vi "test_read-nmea-data2.vi"() -> ()   [LabVIEW 2019] (continued)
248,29,06,64,051,31,6*6C\n\t\n15:15:10.47\tF9P\t$GPGSV,3,2,09,09,44,072,30,12,23,275,18,17,31,154,18,19,51,157,,6*6D\n\t\n15:15:10.49\tF9P\t$GPGSV,3,3,09,25,12,305,,6*58\n\t\n15:15:10.51\tF9P\t$GLGSV,2,1,08,69,10,031,25,70,70,037,29,71,54,207,37,72,05,210,,1*72\n\t\n15:15:10.53\tF9P\t$GLGSV,2,2,08,77,01,324,,84,19,123,16,85,69,072,34,86,38,331,,1*73\n\t\n15:15:10.55\tF9P\t$GLGSV,2,1,08,69,10,031,19,70,70,037,,71,54,207,29,72,05,210,,3*7B\n\t\n15:15:10.57\tF9P\t$GLGSV,2,2,08,77,01,324,,84,19,123,19,85,69,072,27,86,38,331,,3*7C\n\t\n15:15:10.59\tF9P\t$GAGSV,2,1,08,02,08,296,10,04,67,115,41,09,33,193,23,11,72,001,30,7*7F\n\t\n15:15:10.61\tF9P\t$GAGSV,2,2,08,12,39,103,22,19,25,045,28,25,08,248,,36,27,309,22,7*7F\n\t\n15:15:10.63\tF9P\t$GAGSV,2,1,08,02,08,296,,04,67,115,,09,33,193,,11,72,001,,2*7C\n\t\n15:15:10.65\tF9P\t$GAGSV,2,2,08,12,39,103,,19,25,045,20,25,08,248,,36,27,309,,2*72\n\t\n15:15:10.67\tF9P\t$GBGSV,2,1,06,07,,,21,11,48,133,38,14,87,101,28,28,,,24,1*7D\n\t\n15:15:10.69\tF9P\t$GBGSV,2,2,06,33,62,220,29,34,,,28,1*42\n\t\n15:15:10.71\tF9P\t$GBGSV,1,1,03,11,48,133,,14,87,101,28,33,62,220,,3*4E\n\t\n15:15:10.73\tF9P\t$GNGLL,3723.60078,N,12656.94421,E,061512.00,A,A*76\n\t\n15:15:10.75\tF9P\t\t\n15:15:10.77\tF9P\t\t\n15:15:10.79\tF9P\t\t\n15:15:10.81\tF9P\t\t\n15:15:10.83\tF9P\t\t\n15:15:10.85\tF9P\t\t\n15:15:10.87\tF9P\t\t\n15:15:10.89\tF9P\t\t\n15:15:10.91\tF9P\t\t\n15:15:10.93\tF9P\t\t\n15:15:10.95\tF9P\t\t\n15:15:10.97\tF9P\t\t\n15:15:10.99\tF9P\t\t\n15:15:11.01\tF9P\t\t\n15:15:11.03\tF9P\t\t\n15:15:11.05\tF9P\t\t\n15:15:11.07\tF9P\t\t\n15:15:11.09\tF9P\t\t\n15:15:11.11\tF9P\t\t\n15:15:11.13\tF9P\t\t\n15:15:11.15\tF9P\t\t\n15:15:11.17\tF9P\t\t\n15:15:11.19\tF9P\t\t\n15:15:11.21\tF9P\t\t\n15:15:11.23\tF9P\t\t\n15:15:11.25\tF9P\t$GNRMC,061513.00,A,3723.60061,N,12656.94322,E,2.887,256.84,250720,,,A,V*0C\n\t\n15:15:11.27\tF9P\t$GNVTG,256.84,T,,M,2.887,N,5.347,K,A*2E\n\t\n15:15:11.29\tF9P\t$GNGGA,061513.00,3723.60061,N,12656.94322,E,1,12,0.71,45.1,M,18.5,M,,*77\n\t\n15:15:11.31\tF9P\t$GNGSA,A,3,12,06,19,05,17,09,04,02,,,,,1.23,0.71,1.00,1*07\n\t\n15:15:11.33\tF9P\t$GNGSA,A,3,85,70,71,84,,,,,,,,,1.23,0.71,1.00,2*05\n\t\n15:15:11.35\tF9P\t$GNGSA,A,3,36,19,11,04,09,12,,,,,,,1.23,0.71,1.00,3*07\n\t\n15:15:11.37\tF9P\t$GNGSA,A,3,14,11,33,,,,,,,,,,1.23,0.71,1.00,4*06\n\t\n15:15:11.39\tF9P\t$GPGSV,3,1,09,02,56,320,26,04,17,043,29,05,38,248,35,06,64,051,41,1*66\n\t\n15:15:11.41\tF9P\t$GPGSV,3,2,09,09,44,072,39,12,23,275,27,17,31,154,26,19,51,157,27,1*67\n\t\n15:15:11.43\tF9P\t$GPGSV,3,3,09,25,12,305,08,1*57\n\t\n15:15:11.45\tF9P\t$GPGSV,3,1,09,02,56,320,,04,17,043,21,05,38,248,29,06,64,051,31,6*67\n\t\n15:15:11.47\tF9P\t$GPGSV,3,2,09,09,44,072,30,12,23,275,18,17,31,154,17,19,51,157,,6*62\n\t\n15:15:11.49\tF9P\t$GPGSV,3,3,09,25,12,305,,6*58\n\t\n15:15:11.51\tF9P\t$GLGSV,2,1,08,69,10,031,26,70,70,037,29,71,54,207,29,72,05,210,,1*7E\n\t\n15:15:11.53\tF9P\t$GLGSV,2,2,08,77,01,324,,84,19,123,17,85,69,072,34,86,38,331,,1*72\n\t\n15:15:11.55\tF9P\t$GLGSV,2,1,08,69,10,031,19,70,70,037,,71,54,207,28,72,05,210,,3*7A\n\t\n15:15:11.57\tF9P\t$GLGSV,2,2,08,77,01,324,,84,19,123,20,85,69,072,26,86,38,331,,3*77\n\t\n15:15:11.59\tF9P\t$GAGSV,2,1,08,02,08,296,10,04,67,115,40,09,33,193,23,11,72,001,25,7*7A\n\t\n15:15:11.61\tF9P\t$GAGSV,2,2,08,12,39,103,22,19,25,045,29,25,08,248,,36,27,309,29,7*75\n\t\n15:15:11.63\tF9P\t$GAGSV,2,1,08,02,08,296,,04,67,115,29,09,33,193,,11,72,001,,2*77\n\t\n15:15:11.65\tF9P\t$GAGSV,2,2,08,12,39,103,,19,25,045,19,25,08,248,,36,27,309,28,2*72\n\t\n15:15:11.67\tF9P\t$GBGSV,2,1,06,07,,,21,11,48,133,26,14,87,101,28,28,,,24,1*72\n\t\n15:15:11.69\tF9P\t$GBGSV,2,2,06,33,62,220,33,34,,,28,1*49\n\t\n15:15:11.71\tF9P\t$GBGSV,1,1,03,11,48,133,,14,87,101,28,33,62,220,,3*4E\n\t\n15:15:11.73\tF9P\t$GNGLL,3723.60061,N,12656.94322,E,061513.00,A,A*7B\n\t\n15:15:11.75\tF9P\t\t\n15:15:11.77\tF9P\t\t\n15:15:11.79\tF9P\t\t\n15:15:11.81\tF9P\t\t\n15:15:11.83\tF9P\t\t\n15:15:11.85\tF9P\t\t\n15:15:11.87\tF9P\t\t\n15:15:11.89\tF9P\t\t\n15:15:11.91\tF9P\t\t\n15:15:11.93\tF9P\t\t\n15:15:11.95\tF9P\t\t\n15:15:11.97\tF9P\t\t\n15:15:11.99\tF9P\t\t\n15:15:12.01\tF9P\t\t\n15:15:12.03\tF9P\t\t\n15:15:12.05\tF9P\t\t\n15:15:12.07\tF9P\t\t\n15:15:12.09\tF9P\t\t\n15:15:12.11\tF9P\t\t\n15:15:12.13\tF9P\t\t\n15:15:12.15\tF9P\t\t\n15:15:12.17\tF9P\t\t\n15:15:12.19\tF9P\t\t\n15:15:12.21\tF9P\t\t\n15:15:12.23\tF9P\t$GNRMC,061514.00,A,3723.60011,N,12656.94253,E,2.747,249.72,250720,,,A,V*0F\n\t\n15:15:12.25\tF9P\t$GNVTG,249.72,T,,M,2.747,N,5.087,K,A*25\n\t\n15:15:12.27\tF9P\t$GNGGA,061514.00,3723.60011,N,12656.94253,E,1,12,0.75,44.4,M,18.5,M,,*70\n\t\n15:15:12.29\tF9P\t$GNGSA,A,3,12,06,19,05,17,09,04,02,,,,,1.25,0.75,1.01,1*04\n\t\n15:15:12.31\tF9P\t$GNGSA,A,3,85,70,71,84,,,,,,,,,1.25,0.75,1.01,2*06\n\t\n15:15:12.33\tF9P\t$GNGSA,A,3,36,19,11,04,09,12,,,,,,,1.25,0.75,1.01,3*04\n\t\n15:15:12.35\tF9P\t$GNGSA,A,3,14,11,33,,,,,,,,,,1.25,0.75,1.01,4*05\n\t\n15:15:12.37\tF9P\t$GPGSV,3,1,09,02,56,320,26,04,17,043,29,05,38,248,31,06,64,051,40,1*63\n\t\n15:15:12.39\tF9P\t$GPGSV,3,2,09,09,44,072,41,12,23,275,26,17,31,154,27,19,51,157,31,1*6F\n\t\n15:15:12.41\tF9P\t$GPGSV,3,3,09,25,12,305,,1*5F\n\t\n15:15:12.43\tF9P\t$GPGSV,3,1,09,02,56,320,,04,17,043,19,05,38,248,28,06,64,051,32,6*6E\n\t\n15:15:12.45\tF9P\t$GPGSV,3,2,09,09,44,072,29,12,23,275,19,17,31,154,17,19,51,157,,6*6B\n\t\n15:15:12.47\tF9P\t$GPGSV,3,3,09,25,12,305,,6*58\n\t\n15:15:12.49\tF9P\t$GLGSV,2,1,08,69,10,031,31,70,70,037,32,71,54,207,28,72,05,210,,1*73\n\t\n15:15:12.51\tF9P\t$GLGSV,2,2,08,77,01,324,,84,19,123,18,85,69,072,40,86,38,331,,1*7E\n\t\n15:15:12.53\tF9P\t$GLGSV,2,1,08,69,10,031,18,70,70,037,,71,54,207,27,72,05,210,,3*74\n\t\n15:15:12.55\tF9P\t$GLGSV,2,2,08,77,01,324,,84,19,123,21,85,69,072,26,86,38,331,,3*76\n\t\n15:15:12.57\tF9P\t$GAGSV,2,1,08,02,08,296,11,04,67,115,37,09,33,193,30,11,72,001,24,7*78\n\t\n15:15:12.59\tF9P\t$GAGSV,2,2,08,12,39,103,29,19,25,045,33,25,08,248,,36,27,309,27,7*7B\n\t\n15:15:12.61\tF9P\t$GAGSV,2,1,08,02,08,296,,04,67,115,,09,33,193,,11,72,001,,2*7C\n\t\n15:15:12.63\tF9P\t$GAGSV,2,2,08,12,39,103,,19,25,045,19,25,08,248,,36,27,309,25,2*7F\n\t\n15:15:12.65\tF9P\t$GBGSV,2,1,06,07,,,21,11,48,133,27,14,87,101,32,28,,,25,1*79\n\t\n15:15:12.67\tF9P\t$GBGSV,2,2,06,33,62,220,35,34,,,27,1*40\n\t\n15:15:12.69\tF9P\t$GBGSV,1,1,03,11,48,133,,14,87,101,32,33,62,220,,3*45\n\t\n15:15:12.71\tF9P\t$GNGLL,3723.60011,N,12656.94253,E,061514.00,A,A*7C\n\t\n15:15:12.73\tF9P\t\t\n15:15:12.75\tF9P\t\t\n15:15:12.77\tF9P\t\t\n15:15:12.79\tF9P\t\t\n15:15:12.81\tF9P\t\t\n15:15:12.83\tF9P\t\t\n15:15:12.85\tF9P\t\t\n15:15:12.87\tF9P\t\t\n15:15:12.89\tF9P\t\t\n15:15:12.91\tF9P\t\t\n15:15:12.93\tF9P\t\t\n15:15:12.95\tF9P\t\t\n15:15:12.97\tF9P\t\t\n15:15:12.99\tF9P\t\t\n15:15:13.01\tF9P\t\t\n15:15:13.03\tF9P\t\t\n15:15:13.05\tF9P\t\t\n15:15:13.07\tF9P\t\t\n15:15:13.09\tF9P\t\t\n15:15:13.11\tF9P\t\t\n15:15:13.13\tF9P\t\t\n15:15:13.15\tF9P\t\t\n15:15:13.17\tF9P\t\t\n15:15:13.19\tF9P\t\t\n15:15:13.21\tF9P\t\t\n15:15:13.23\tF9P\t$GNRMC,061515.00,A,3723.59977,N,12656.94169,E,2.605,246.33,250720,,,A,V*0A\n\t\n15:15:13.25\tF9P\t$GNVTG,246.33,T,,M,2.605,N,4.825,K,A*29\n\t\n15:15:13.27\tF9P\t$GNGGA,061515.00,3723.59977,N,12656.94169,E,1,12,0.72,44.4,M,18.5,M,,*7F\n\t\n15:15:13.29\tF9P\t$GNGSA,A,3,12,06,19,05,17,09,04,02,,,,,1.24,0.72,1.00,1*03\n\t\n15:15:13.31\tF9P\t$GNGSA,A,3,85,70,71,84,,,,,,,,,1.24,0.72,1.00,2*01\n\t\n15:15:13.33\tF9P\t$GNGSA,A,3,36,19,11,04,09,12,,,,,,,1.24,0.72,1.00,3*03\n\t\n15:15:13.35\tF9P\t$GNGSA,A,3,14,11,33,,,,,,,,,,1.24,0.72,1.00,4*02\n\t\n15:15:13.37\tF9P\t$GPGSV,3,1,09,02,56,320,26,04,17,043,28,05,38,248,34,06,64,051,34,1*64\n\t\n15:15:13.39\tF9P\t$GPGSV,3,2,09,09,44,072,42,12,23,275,27,17,31,154,27,19,51,157,39,1*65\n\t\n15:15:13.41\tF9P\t$GPGSV,3,3,09,25,12,305,,1*5F\n\t\n15:15:13.43\tF9P\t$GPGSV,3,1,09,02,56,320,,04,17,043,20,05,38,248,27,06,64,051,31,6*68\n\t\n15:15:13.45\tF9P\t$GPGSV,3,2,09,09,44,072,31,12,23,275,18,17,31,154,17,19,51,157,,6*63\n\t\n15:15:13.47\tF9P\t$GPGSV,3,3,09,25,12,305,,6*58\n\t\n15:15:13.49\tF9P\t$GLGSV,2,1,08,69,10,031,31,70,70,037,25,71,54,207,36,72,05,210,,1*7A\n\t\n15:15:13.51\tF9P\t$GLGSV,2,2,08,77,01,324,,84,19,123,18,85,69,072,36,86,38,331,,1*7F\n\t\n15:15:13.53\tF9P\t$GLGSV,2,1,08,69,10,031,17,70,70,037,,71,54,207,25,72,05,210,,3*79\n\t\n15:15:13.55\tF9P\t$GLGSV,2,2,08,77,01,324,,84,19,123,19,85,69,072,27,86,38,331,,3*7C\n\t\n15:15:13.57\tF9P\t$GAGSV,2,1,08,02,08,296,09,04,67,115,37,09,33,193,30,11,72,001,25,7*70\n\t\n15:15:13.59\tF9P\t$GAGSV,2,2,08,12,39,103,27,19,25,045,28,25,08,248,,36,27,309,25,7*7D\n\t\n15:15:13.61\tF9P\t$GAGSV,2,1,08,02,08,296,,04,67,115,,09,33,193,,11,72,001,,2*7C\n\t\n15:15:13.63\tF9P\t$GAGSV,2,2,08,12,39,103,,19,25,045,20,25,08,248,,36,27,309,23,2*73\n\t\n15:15:13.65\tF9P\t$GBGSV,2,1,06,07,,,21,11,48,133,32,14,87,101,32,28,,,31,1*78\n\t\n15:15:13.67\tF9P\t$GBGSV,2,2,06,33,62,220,36,34,,,27,1*43\n\t\n15:15:13.69\tF9P\t$GBGSV,1,1,03,11,48,133,,14,87,101,29,33,62,220,,3*4F\n\t\n15:15:13.71\tF9P\t$GNGLL,3723.59977,N,12656.94169,E,061515.00,A,A*74\n\t\n15:15:13.73\tF9P\t\t\n15:15:13.75\tF9P\t\t\n15:15:13.77\tF9P\t\t\n15:15:13.79\tF9P\t\t\n15:15:13.81\tF9P\t\t\n15:15:13.83\tF9P\t\t\n15:15:13.85\tF9P\t\t\n15:15:13.87\tF9P\t\t\n15:15:13.89\tF9P\t\t\n15:15:13.91\tF9P\t\t\n15:15:13.93\tF9P\t\t\n15:15:13.95\tF9P\t\t\n15:15:13.97\tF9P\t\t\n15:15:13.99\tF9P\t\t\n15:15:14.01\tF9P\t\t\n15:15:14.03\tF9P\t\t\n15:15:14.05\tF9P\t\t\n15:15:14.07\tF9P\t\t\n15:15:14.09\tF9P\t\t\n15:15:14.11\tF9P\t\t\n15:15:14.13\tF9P\t\t\n15:15:14.15\tF9P\t\t\n15:15:14.17\tF9P\t\t\n15:15:14.19\tF9P\t\t\n15:15:14.21\tF9P\t\t\n15:15:14.23\tF9P\t\t\n15:15:14.25\tF9P\t$GNRMC,061516.00,A,3723.59953,N,12656.94080,E,2.577,247.44,250720,,,A,V*0E\n\t\n15:15:14.27\tF9P\t$GNVTG,247.44,T,,M,2.577,N,4.773,K,A*22\n\t\n15:15:14.29\tF9P\t$GNGGA,061516.00,3723.59953,N,12656.94080,E,1,12,0.67,44.5,M,18.5,M,,*79\n\t\n15:15:14.31\tF9P\t$GNGSA,A,3,12,06,19,05,17,09,04,02,,,,,1.18,0.67,0.97,1*07\n\t\n15:15:14.33\tF9P\t$GNGSA,A,3,85,70,71,84,,,,,,,,,1.18,0.67,0.97,2*05\n\t\n15:15:14.35\tF9P\t$GNGSA,A,3,36,19,11,04,09,12,,,,,,,1.18,0.67,0.97,3*07\n\t\n15:15:14.37\tF9P\t$GNGSA,A,3,14,11,33,,,,,,,,,,1.18,0.67,0.97,4*06\n\t\n15:15:14.39\tF9P\t$GPGSV,3,1,09,02,56,320,27,04,17,043,32,05,38,248,35,06,64,051,38,1*63\n\t\n15:15:14.41\tF9P\t$GPGSV,3,2,09,09,44,072,43,12,23,275,28,17,31,154,37,19,51,157,36,1*65\n\t\n15:15:14.43\tF9P\t$GPGSV,3,3,09,25,12,305,,1*5F\n\t\n15:15:14.45\tF9P\t$GPGSV,3,1,09,02,56,320,,04,17,043,20,05,38,248,27,06,64,051,32,6*6B\n\t\n15:15:14.47\tF9P\t$GPGSV,3,2,09,09,44,072,32,12,23,275,19,17,31,154,19,19,51,157,,6*6F\n\t\n15:15:14.49\tF9P\t$GPGSV,3,3,09,25,12,305,,6*58\n\t\n15:15:14.51\tF9P\t$GLGSV,2,1,08,69,10,031,26,70,70,037,31,71,54,207,28,72,05,210,,1*76\n\t\n15:15:14.53\tF9P\t$GLGSV,2,2,08,77,01,324,,84,19,123,17,85,69,072,41,86,38,331,,1*70\n\t\n15:15:14.55\tF9P\t$GLGSV,2,1,08,69,10,031,17,70,70,037,,71,54,207,25,72,05,210,,3*79\n\t\n15:15:14.57\tF9P\t$GLGSV,2,2,08,77,01,324,,84,19,123,20,85,69,072,27,86,38,331,,3*76\n\t\n15:15:14.59\tF9P\t$GAGSV,2,1,08,02,08,296,10,04,67,115,33,09,33,193,28,11,72,001,23,7*73\n\t\n15:15:14.61\tF9P\t$GAGSV,2,2,08,12,39,103,19,19,25,045,28,25,08,248,,36,27,309,24,7*71\n\t\n15:15:14.63\tF9P\t$GAGSV,2,1,08,02,08,296,,04,67,115,,09,33,193,,11,72,001,,2*7C\n\t\n15:15:14.65\tF9P\t$GAGSV,2,2,08,12,39,103,,19,25,045,19,25,08,248,,36,27,309,19,2*70\n\t\n15:15:14.67\tF9P\t$GBGSV,2,1,06,07,,,23,11,48,133,26,14,87,101,32,28,,,26,1*79\n\t\n15:15:14.69\tF9P\t$GBGSV,2,2,06,33,62,220,36,34,,,27,1*43\n\t\n15:15:14.71\tF9P\t$GBGSV,1,1,03,11,48,133,,14,87,101,29,33,62,220,,3*4F\n\t\n15:15:14.73\tF9P\t$GNGLL,3723.59953,N,12656.94080,E,061516.00,A,A*77\n\t\n15:15:14.75\tF9P\t\t\n15:15:14.77\tF9P\t\t\n15:15:14.79\tF9P\t\t\n15:15:14.81\tF9P\t\t\n15:15:14.83\tF9P\t\t\n15:15:14.85\tF9P\t\t\n15:15:14.87\tF9P\t\t\n15:15:14.89\tF9P\t\t\n15:15:14.91\tF9P\t\t\n15:15:14.93\tF9P\t\t\n15:15:14.95\tF9P\t\t\n15:15:14.97\tF9P\t\t\n15:15:14.99\tF9P\t\t\n15:15:15.01\tF9P\t\t\n15:15:15.03\tF9P\t\t\n15:15:15.05\tF9P\t\t\n15:15:15.07\tF9P\t\t\n15:15:15.09\tF9P\t\t\n15:15:15.11\tF9P\t\t\n15:15:15.13\tF9P\t\t\n15:15:15.15\tF9P\t\t\n15:15:15.17\tF9P\t\t\n15:15:15.19\tF9P\t\t\n15:15:15.21\tF9P\t\t\n15:15:15.23\tF9P\t$GNRMC,061517.00,A,3723.59946,N,12656.93983,E,2.372,251.56,250720,,,A,V*01\n\t\n15:15:15.25\tF9P\t$GNVTG,251.56,T,,M,2.372,N,4.393,K,A*2F\n\t\n15:15:15.27\tF9P\t$GNGGA,061517.00,3723.59946,N,12656.93983,E,1,12,0.68,45.3,M,18.5,M,,*79\n\t\n15:15:15.29\tF9P\t$GNGSA,A,3,12,06,19,05,17,09,04,02,,,,,1.20,0.68,0.98,1*0C\n\t\n15:15:15.31\tF9P\t$GNGSA,A,3,85,70,71,84,,,,,,,,,1.20,0.68,0.98,2*0E\n\t\n15:15:15.33\tF9P\t$GNGSA,A,3,36,19,11,04,09,12,,,,,,,1.20,0.68,0.98,3*0C\n\t\n15:15:15.35\tF9P\t$GNGSA,A,3,14,11,33,,,,,,,,,,1.20,0.68,0.98,4*0D\n\t\n15:15:15.37\tF9P\t$GPGSV,3,1,09,02,56,320,27,04,17,043,26,05,38,248,36,06,64,051,41,1*6B\n\t\n15:15:15.39\tF9P\t$GPGSV,3,2,09,09,44,072,41,12,23,275,29,17,31,154,42,19,51,157,35,1*67\n\t\n15:15:15.41\tF9P\t$GPGSV,3,3,09,25,12,305,,1*5F\n\t\n15:15:15.43\tF9P\t$GPGSV,3,1,09,02,56,320,,04,17,043,20,05,38,248,27,06,64,051,31,6*68\n\t\n15:15:15.45\tF9P\t$GPGSV,3,2,09,09,44,072,33,12,23,275,18,17,31,154,20,19,51,157,,6*65\n\t\n15:15:15.47\tF9P\t$GPGSV,3,3,09,25,12,305,,6*58\n\t\n15:15:15.49\tF9P\t$GLGSV,2,1,08,69,10,031,31,70,70,037,32,71,54,207,28,72,05,210,,1*73\n\t\n15:15:15.51\tF9P\t$GLGSV,2,2,08,77,01,324,,84,19,123,16,85,69,072,44,86,38,331,,1*74\n\t\n15:15:15.53\tF9P\t$GLGSV,2,1,08,69,10,031,17,70,70,037,,71,54,207,24,72,05,210,,3*78\n\t\n15:15:15.55\tF9P\t$GLGSV,2,2,08,77,01,324,,84,19,123,21,85,69,072,27,86,38,331,,3*77\n\t\n15:15:15.57\tF9P\t$GAGSV,2,1,08,02,08,296,10,04,67,115,35,09,33,193,28,11,72,001,24,7*72\n\t\n15:15:15.59\tF9P\t$GAGSV,2,2,08,12,39,103,23,19,25,045,28,25,08,248,,36,27,309,23,7*7F\n\t\n15:15:15.61\tF9P\t$GAGSV,2,1,08,02,08,296,,04,67,115,,09,33,193,,11,72,001,,2*7C\n\t\n15:15:15.63\tF9P\t$GAGSV,2,2,08,12,39,103,,19,25,045,20,25,08,248,,36,27,309,18,2*7B\n\t\n15:15:15.65\tF9P\t$GBGSV,2,1,06,07,,,24,11,48,133,27,14,87,101,29,28,,,26,1*75\n\t\n15:15:15.67\tF9P\t$GBGSV,2,2,06,33,62,220,34,34,,,26,1*40\n\t\n15:15:15.69\tF9P\t$GBGSV,1,1,03,11,48,133,,14,87,101,34,33,62,220,,3*43\n\t\n15:15:15.71\tF9P\t$GNGLL,3723.59946,N,12656.93983,E,061517.00,A,A*7F\n\t\n15:15:15.73\tF9P\t\t\n15:15:15.75\tF9P\t\t\n15:15:15.77\tF9P\t\t\n15:15:15.79\tF9P\t\t\n15:15:15.81\tF9P\t\t\n15:15:15.83\tF9P\t\t\n15:15:15.85\tF9P\t\t\n15:15:15.87\tF9P\t\t\n15:15:15.89\tF9P\t\t\n15:15:15.91\tF9P\t\t\n15:15:15.93\tF9P\t\t\n15:15:15.95\tF9P\t\t\n15:15:15.97\tF9P\t\t\n15:15:15.99\tF9P\t\t\n15:15:16.01\tF9P\t\t\n15:15:16.03\tF9P\t\t\n15:15:16.05\tF9P\t\t\n15:15:16.07\tF9P\t\t\n15:15:16.09\tF9P\t\t\n15:15:16.11\tF9P\t\t\n15:15:16.13\tF9P\t\t\n15:15:16.15\tF9P\t\t\n15:15:16.17\tF9P\t\t\n15:15:16.19\tF9P\t\t\n15:15:16.21\tF9P\t\t\n15:15:16.23\tF9P\t$GNRMC,061518.00,A,3723.59925,N,12656.93903,E,2.550,252.52,250720,,,A,V*02\n\t\n15:15:16.25\tF9P\t$GNVTG,252.52,T,,M,2.550,N,4.723,K,A*21\n\t\n15:15:16.27\tF9P\t$GNGGA,061518.00,3723.59925,N,12656.93903,E,1,12,0.66,45.8,M,18.5,M,,*7E\n\t\n15:15:16.29\tF9P\t$GNGSA,A,3,12,06,19,05,17,09,04,02,,,,,1.15,0.66,0.94,1*08\n\t\n15:15:16.31\tF9P\t$GNGSA,A,3,85,70,71,84,,,,,,,,,1.15,0.66,0.94,2*0A\n\t\n15:15:16.33\tF9P\t$GNGSA,A,3,36,19,11,04,09,12,,,,,,,1.15,0.66,0.94,3*08\n\t\n15:15:16.35\tF9P\t$GNGSA,A,3,14,11,33,,,,,,,,,,1.15,0.66,0.94,4*09\n\t\n15:15:16.37\tF9P\t$GPGSV,3,1,09,02,56,320,35,04,17,043,28,05,38,248,38,06,64,051,35,1*6B\n\t\n15:15:16.39\tF9P\t$GPGSV,3,2,09,09,44,072,42,12,23,275,28,17,31,154,38,19,51,157,36,1*6B\n\t\n15:15:16.41\tF9P\t$GPGSV,3,3,09,25,12,305,,1*5F\n\t\n15:15:16.43\tF9P\t$GPGSV,3,1,09,02,56,320,,04,17,043,20,05,38,248,25,06,64,051,31,6*6A\n\t\n15:15:16.45\tF9P\t$GPGSV,3,2,09,09,44,072,32,12,23,275,18,17,31,154,21,19,51,157,,6*65\n\t\n15:15:16.47\tF9P\t$GPGSV,3,3,09,25,12,305,,6*58\n\t\n15:15:16.49\tF9P\t$GLGSV,2,1,08,69,10,031,24,70,70,037,32,71,54,207,32,72,05,210,,1*7C\n\t\n15:15:16.51\tF9P\t$GLGSV,2,2,08,77,01,324,,84,19,123,16,85,69,072,44,86,38,331,,1*74\n\t\n15:15:16.53\tF9P\t$GLGSV,2,1,08,69,10,031,17,70,70,037,,71,54,207,23,72,05,210,,3*7F\n\t\n15:15:16.55\tF9P\t$GLGSV,2,2,08,77,01,324,,84,19,123,22,85,69,072,27,86,38,331,,3*74\n\t\n15:15:16.57\tF9P\t$GAGSV,2,1,08,02,08,296,17,04,67,115,32,09,33,193,32,11,72,001,24,7*79\n\t\n15:15:16.59\tF9P\t$GAGSV,2,2,08,12,39,103,25,19,25,045,20,25,08,248,,36,27,309,25,7*77\n\t\n15:15:16.61\tF9P\t$GAGSV,2,1,08,02,08,296,,04,67,115,,09,33,193,,11,72,001,,2*7C\n\t\n15:15:16.63\tF9P\t$GAGSV,2,2,08,12,39,103,,19,25,045,19,25,08,248,,36,27,309,17,2*7E\n\t\n15:15:16.65\tF9P\t$GBGSV,2,1,06,07,,,24,11,48,133,25,14,87,101,36,28,,,26,1*79\n\t\n15:15:16.67\tF9P\t$GBGSV,2,2,06,33,62,220,35,34,,,25,1*42\n\t\n15:15:16.69\tF9P\t$GBGSV,1,1,03,11,48,133,,14,87,101,33,33,62,220,,3*44\n\t\n15:15:16.71\tF9P\t$GNGLL,3723.59925,N,12656.93903,E,061518.00,A,A*7D\n\t\n15:15:16.73\tF9P\t\t\n15:15:16.75\tF9P\t\t\n15:15:16.77\tF9P\t\t\n15:15:16.79\tF9P\t\t\n15:15:16.81\tF9P\t\t\n15:15:16.83\tF9P\t\t\n15:15:16.85\tF9P\t\t\n15:15:16.87\tF9P\t\t\n15:15:16.89\tF9P\t\t\n15:15:16.91\tF9P\t\t\n15:15:16.93\tF9P\t\t\n15:15:16.95\tF9P\t\t\n15:15:16.97\tF9P\t\t\n15:15:16.99\tF9P\t\t\n15:15:17.01\tF9P\t\t\n15:15:17.03\tF9P\t\t\n15:15:17.05\tF9P\t\t\n15:15:17.07\tF9P\t\t\n15:15:17.09\tF9P\t\t\n15:15:17.11\tF9P\t\t\n15:15:17.13\tF9P\t\t\n15:15:17.15\tF9P\t\t\n15:15:17.17\tF9P\t\t\n15:15:17.19\tF9P\t\t\n15:15:17.21\tF9P\t\t\n15:15:17.23\tF9P\t$GNRMC,061519.00,A,3723.59899,N,12656.93822,E,2.579,248.97,250720,,,A,V*0E\n\t\n15:15:17.25\tF9P\t$GNVTG,248.97,T,,M,2.579,N,4.777,K,A*29\n\t\n15:15:17.27\tF9P\t$GNGGA,061519.00,3723.59899,N,12656.93822,E,1,12,0.65,45.9,M,18.5,M,,*79\n\t\n15:15:17.29\tF9P\t$GNGSA,A,3,12,06,19,05,17,09,04,02,,,,,1.14,0.65,0.94,1*0A\n\t\n15:15:17.31\tF9P\t$GNGSA,A,3,85,70,71,84,,,,,,,,,1.14,0.65,0.94,2*08\n\t\n15:15:17.33\tF9P\t$GNGSA,A,3,36,19,11,04,09,12,,,,,,,1.14,0.65,0.94,3*0A\n\t\n15:15:17.35\tF9P\t$GNGSA,A,3,14,11,33,,,,,,,,,,1.14,0.65,0.94,4*0B\n\t\n15:15:17.37\tF9P\t$GPGSV,3,1,09,02,56,320,32,04,17,043,35,05,38,248,30,06,64,051,32,1*6F\n\t\n15:15:17.39\tF9P\t$GPGSV,3,2,09,09,44,072,43,12,23,275,33,17,31,154,35,19,51,157,29,1*63\n\t\n15:15:17.41\tF9P\t$GPGSV,3,3,09,25,12,305,19,1*57\n\t\n15:15:17.43\tF9P\t$GPGSV,3,1,09,02,56,320,,04,17,043,22,05,38,248,27,06,64,051,32,6*69\n\t\n15:15:17.45\tF9P\t$GPGSV,3,2,09,09,44,072,34,12,23,275,18,17,31,154,22,19,51,157,,6*60\n\t\n15:15:17.47\tF9P\t$GPGSV,3,3,09,25,12,305,,6*58\n\t\n15:15:17.49\tF9P\t$GLGSV,2,1,08,69,10,031,31,70,70,037,32,71,54,207,28,72,05,210,,1*73\n\t\n15:15:17.51\tF9P\t$GLGSV,2,2,08,77,01,324,,84,19,123,15,85,69,072,43,86,38,331,,1*70\n\t\n15:15:17.53\tF9P\t$GLGSV,2,1,08,69,10,031,19,70,70,037,,71,54,207,25,72,05,210,,3*77\n\t\n15:15:17.55\tF9P\t$GLGSV,2,2,08,77,01,324,,84,19,123,20,85,69,072,26,86,38,331,,3*77\n\t\n15:15:17.57\tF9P\t$GAGSV,2,1,08,02,08,296,10,04,67,114,31,09,33,193,32,11,72,001,24,7*7C\n\t\n15:15:17.59\tF9P\t$GAGSV,2,2,08,12,39,103,31,19,25,045,30,25,08,248,,36,27,309,23,7*75\n\t\n15:15:17.61\tF9P\t$GAGSV,2,1,08,02,08,296,,04,67,114,,09,33,193,21,11,72,001,,2*7E\n\t\n15:15:17.63\tF9P\t$GAGSV,2,2,08,12,39,103,,19,25,045,20,25,08,248,,36,27,309,19,2*7A\n\t\n15:15:17.65\tF9P\t$GBGSV,2,1,06,07,,,23,11,48,133,27,14,87,101,33,28,,,26,1*79\n\t\n15:15:17.67\tF9P\t$GBGSV,2,2,06,33,62,220,30,34,,,26,1*44\n\t\n15:15:17.69\tF9P\t$GBGSV,1,1,03,11,48,133,,14,87,101,34,33,62,220,,3*43\n\t\n15:15:17.71\tF9P\t$GNGLL,3723.59899,N,12656.93822,E,061519.00,A,A*78\n\t\n15:15:17.74\tF9P\t\t\n15:15:17.76\tF9P\t\t\n15:15:17.78\tF9P\t\t\n15:15:17.80\tF9P\t\t\n15:15:17.82\tF9P\t\t\n15:15:17.84\tF9P\t\t\n15:15:17.86\tF9P\t\t\n15:15:17.88\tF9P\t\t\n15:15:17.90\tF9P\t\t\n15:15:17.92\tF9P\t\t\n15:15:17.94\tF9P\t\t\n15:15:17.96\tF9P\t\t\n15:15:17.98\tF9P\t\t\n15:15:18.00\tF9P\t\t\n15:15:18.02\tF9P\t\t\n15:15:18.04\tF9P\t\t\n15:15:18.06\tF9P\t\t\n15:15:18.08\tF9P\t\t\n15:15:18.10\tF9P\t\t\n15:15:18.12\tF9P\t\t\n15:15:18.14\tF9P\t\t\n15:15:18.16\tF9P\t\t\n15:15:18.18\tF9P\t\t\n15:15:18.20\tF9P\t\t\n
